vi "AlGaInPAs_v20a.vi"(2 "Debug Mode":bool, 3 "Elapsed Time(s)":dbl, 4 "State":enum16{"Edit", "Start", "Run", "End", "Idle"}(ring), 5 "Argument List In":string[](array[string])) -> (0 "Status Out":string, 1 "Argument List Out":string[](array[string]))   [LabVIEW 2011]
uses:
  high_level_proc/Al_bubbler.ctl
  high_level_proc/bubblerDilution.ctl
  high_level_proc/In_bubbler.ctl
  high_level_proc/P_gas.ctl
  high_level_proc/As_gas.ctl
  high_level_proc/P_bubbler.ctl
panel:
  out "Se bubbler Copy":T1={"Active"=FALSE, "main"={"Flow"=0.0, "Run"=FALSE, "Prep Ga"=FALSE, "Dilution"=FALSE, "Calculated"=1, "MFC2 flow"=10.0, "MFC3 flow"=100.0, "MFC1 flow"=0.0}} {"main"."MFC1 flow" format="%.4f"; "main"."MFC3 flow" format="%.1f"; "main"."MFC2 flow" format="%.2f"; "main"."Calculated" items=["Ga flow", "MFC1", "MFC2", "MFC3"]; "main"."Flow" format="%.2f"}
  in  "Se bubbler":T1={"Active"=FALSE, "main"={"Flow"=0.0, "Run"=FALSE, "Prep Ga"=FALSE, "Dilution"=FALSE, "Calculated"=0, "MFC2 flow"=10.0, "MFC3 flow"=100.0, "MFC1 flow"=0.0}} {"main"."MFC1 flow" format="%.4f"; "main"."MFC3 flow" format="%.1f"; "main"."MFC2 flow" format="%.2f"; "main"."Calculated" items=["Flow", "MFC1", "MFC2", "MFC3"]; "main"."Flow" format="%.2f"}
  out "P bubbler Copy":T2 {"P bubbler main"."Flow" format="%.2f"}
  in  "P bubbler":T3 {"P bubbler main"."Flow" format="%.2f"}
  out "As gas Copy":T4 {"As gas main"."Flow" format="%.2f"}
  in  "As gas":T5 {"As gas main"."Flow" format="%.2f"}
  out "P gas Copy":T6 {"P gas main"."Flow" format="%.2f"}
  in  "P gas":T7 {"P gas main"."Flow" format="%.2f"}
  out "In bubbler Copy":T8 {"In main"."Flow" format="%.2f"}
  in  "In bubbler":T9 {"In main"."Flow" format="%.2f"}
  out "Ga bubbler Copy":T10={"Ga bubbler Active"=FALSE, "Ga main"={"Flow"=0.0, "Ga Run"=FALSE, "Prep Ga"=FALSE, "Dilution"=FALSE, "Ga Calculated"=1, "MFC2 flow"=10.0, "MFC3 flow"=100.0, "MFC1 flow"=0.0}} {"Ga main"."MFC1 flow" format="%.4f"; "Ga main"."MFC3 flow" format="%.1f"; "Ga main"."MFC2 flow" format="%.2f"; "Ga main"."Ga Calculated" items=["Ga flow", "MFC1", "MFC2", "MFC3"]; "Ga main"."Flow" format="%.2f"}
  in  "Ga bubbler":T1={"Active"=FALSE, "main"={"Flow"=0.0, "Run"=FALSE, "Prep Ga"=FALSE, "Dilution"=FALSE, "Calculated"=0, "MFC2 flow"=10.0, "MFC3 flow"=100.0, "MFC1 flow"=0.0}} {"main"."MFC1 flow" format="%.4f"; "main"."MFC3 flow" format="%.1f"; "main"."MFC2 flow" format="%.2f"; "main"."Calculated" items=["Flow", "MFC1", "MFC2", "MFC3"]; "main"."Flow" format="%.2f"}
  out "Al bubbler Copy":T11 {"Al main"."Al Flow" format="%.2f"}
  in  "Al bubbler":T12 {"Al main"."Al Flow" format="%.2f"}
  out "prep_done":bool
  out "run started":bool
  out "first":bool=TRUE
  out "total time":dbl
  out "is OK?":bool
  in  "prep_time":dbl
  in  "Cancel":bool
  in  "OK":bool
  out "tTotal(s) 2":dbl
  # "s"
  # "Add pre-run time to run time in editor."
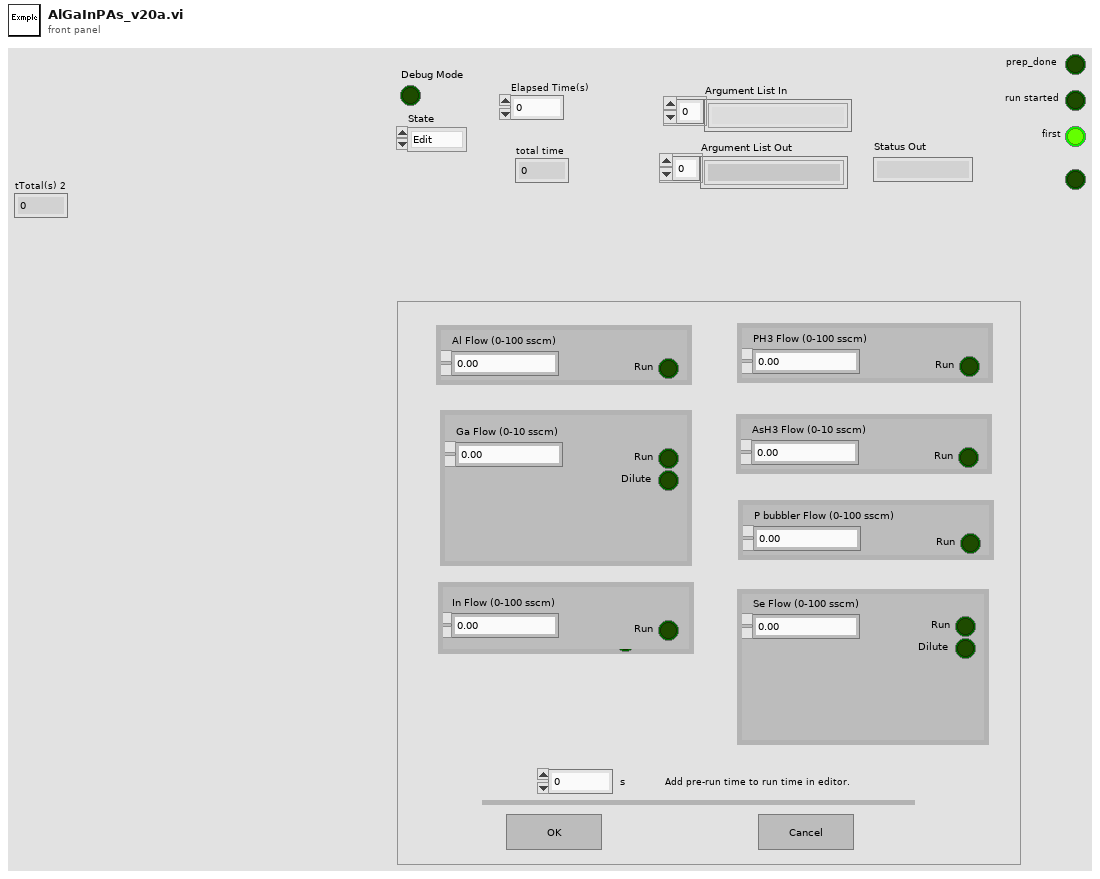
[diagram p1: front panel]
types:
  T1 = typedef "bubblerDilution.ctl" = cluster{"Active":bool, "main":cluster{"Flow":dbl, "Run":bool, "Prep Ga":bool, "Dilution":bool, "Calculated":u16, "MFC2 flow":dbl, "MFC3 flow":dbl, "MFC1 flow":dbl}}
  T2 = cluster{"P bubbler Active":bool, "P bubbler main":cluster{"Flow":dbl, "P bubbler Run":bool, "P bubbler Prep":bool}}
  T3 = typedef "P_bubbler.ctl" = cluster{"P bubbler Active":bool, "P bubbler main":cluster{"Flow":dbl, "P bubbler Run":bool, "P bubbler Prep":bool}}
  T4 = cluster{"As gas Active":bool, "As gas main":cluster{"Flow":dbl, "AsH3 Run":bool, "AsH3 Prep":bool}}
  T5 = typedef "As_gas.ctl" = cluster{"As gas Active":bool, "As gas main":cluster{"Flow":dbl, "AsH3 Run":bool, "AsH3 Prep":bool}}
  T6 = cluster{"P gas Active":bool, "P gas main":cluster{"Flow":dbl, "PH3 Run":bool, "PH3 Prep":bool}}
  T7 = typedef "P_gas.ctl" = cluster{"P gas Active":bool, "P gas main":cluster{"Flow":dbl, "PH3 Run":bool, "PH3 Prep":bool}}
  T8 = cluster{"In main":cluster{"Flow":dbl, "In Run":bool, "Prep In":bool}, "In bubbler Active":bool}
  T9 = typedef "In_bubbler.ctl" = cluster{"In main":cluster{"Flow":dbl, "In Run":bool, "Prep In":bool}, "In bubbler Active":bool}
  T10 = cluster{"Ga bubbler Active":bool, "Ga main":cluster{"Flow":dbl, "Ga Run":bool, "Prep Ga":bool, "Dilution":bool, "Ga Calculated":u16, "MFC2 flow":dbl, "MFC3 flow":dbl, "MFC1 flow":dbl}}
  T11 = cluster{"Al Active":bool, "Al main":cluster{"Al Flow":dbl, "Al Run":bool, "Prep Al":bool}}
  T12 = typedef "Al_bubbler.ctl" = cluster{"Al Active":bool, "Al main":cluster{"Al Flow":dbl, "Al Run":bool, "Prep Al":bool}}
  T13 = enum16{"Discrete", "Continuous", "Instantaneous", "Finite"}
  T14 = enum32{"Invalid", "Default", "Floating", "Floating/Auto-Hide", "Modal"}
  T15 = enum8{"Enabled", "Disabled", "Disabled and Grayed Out"}
  T16 = cluster{"Active":bool, "main":cluster{"Flow":dbl, "Run":bool, "Prep Ga":bool, "Dilution":bool, "Calculated":u16, "MFC2 flow":dbl, "MFC3 flow":dbl, "MFC1 flow":dbl}}
  T17 = cluster{"Al Flow":dbl, "Al Run":bool, "Prep Al":bool}
  T18 = cluster{"Flow":dbl, "Run":bool, "Prep Ga":bool, "Dilution":bool, "Calculated":u16, "MFC2 flow":dbl, "MFC3 flow":dbl, "MFC1 flow":dbl}
  T19 = cluster{"Flow":dbl, "In Run":bool, "Prep In":bool}
  T20 = cluster{"Flow":dbl, "PH3 Run":bool, "PH3 Prep":bool}
  T21 = cluster{"Flow":dbl, "AsH3 Run":bool, "AsH3 Prep":bool}
  T22 = cluster{"Flow":dbl, "P bubbler Run":bool, "P bubbler Prep":bool}
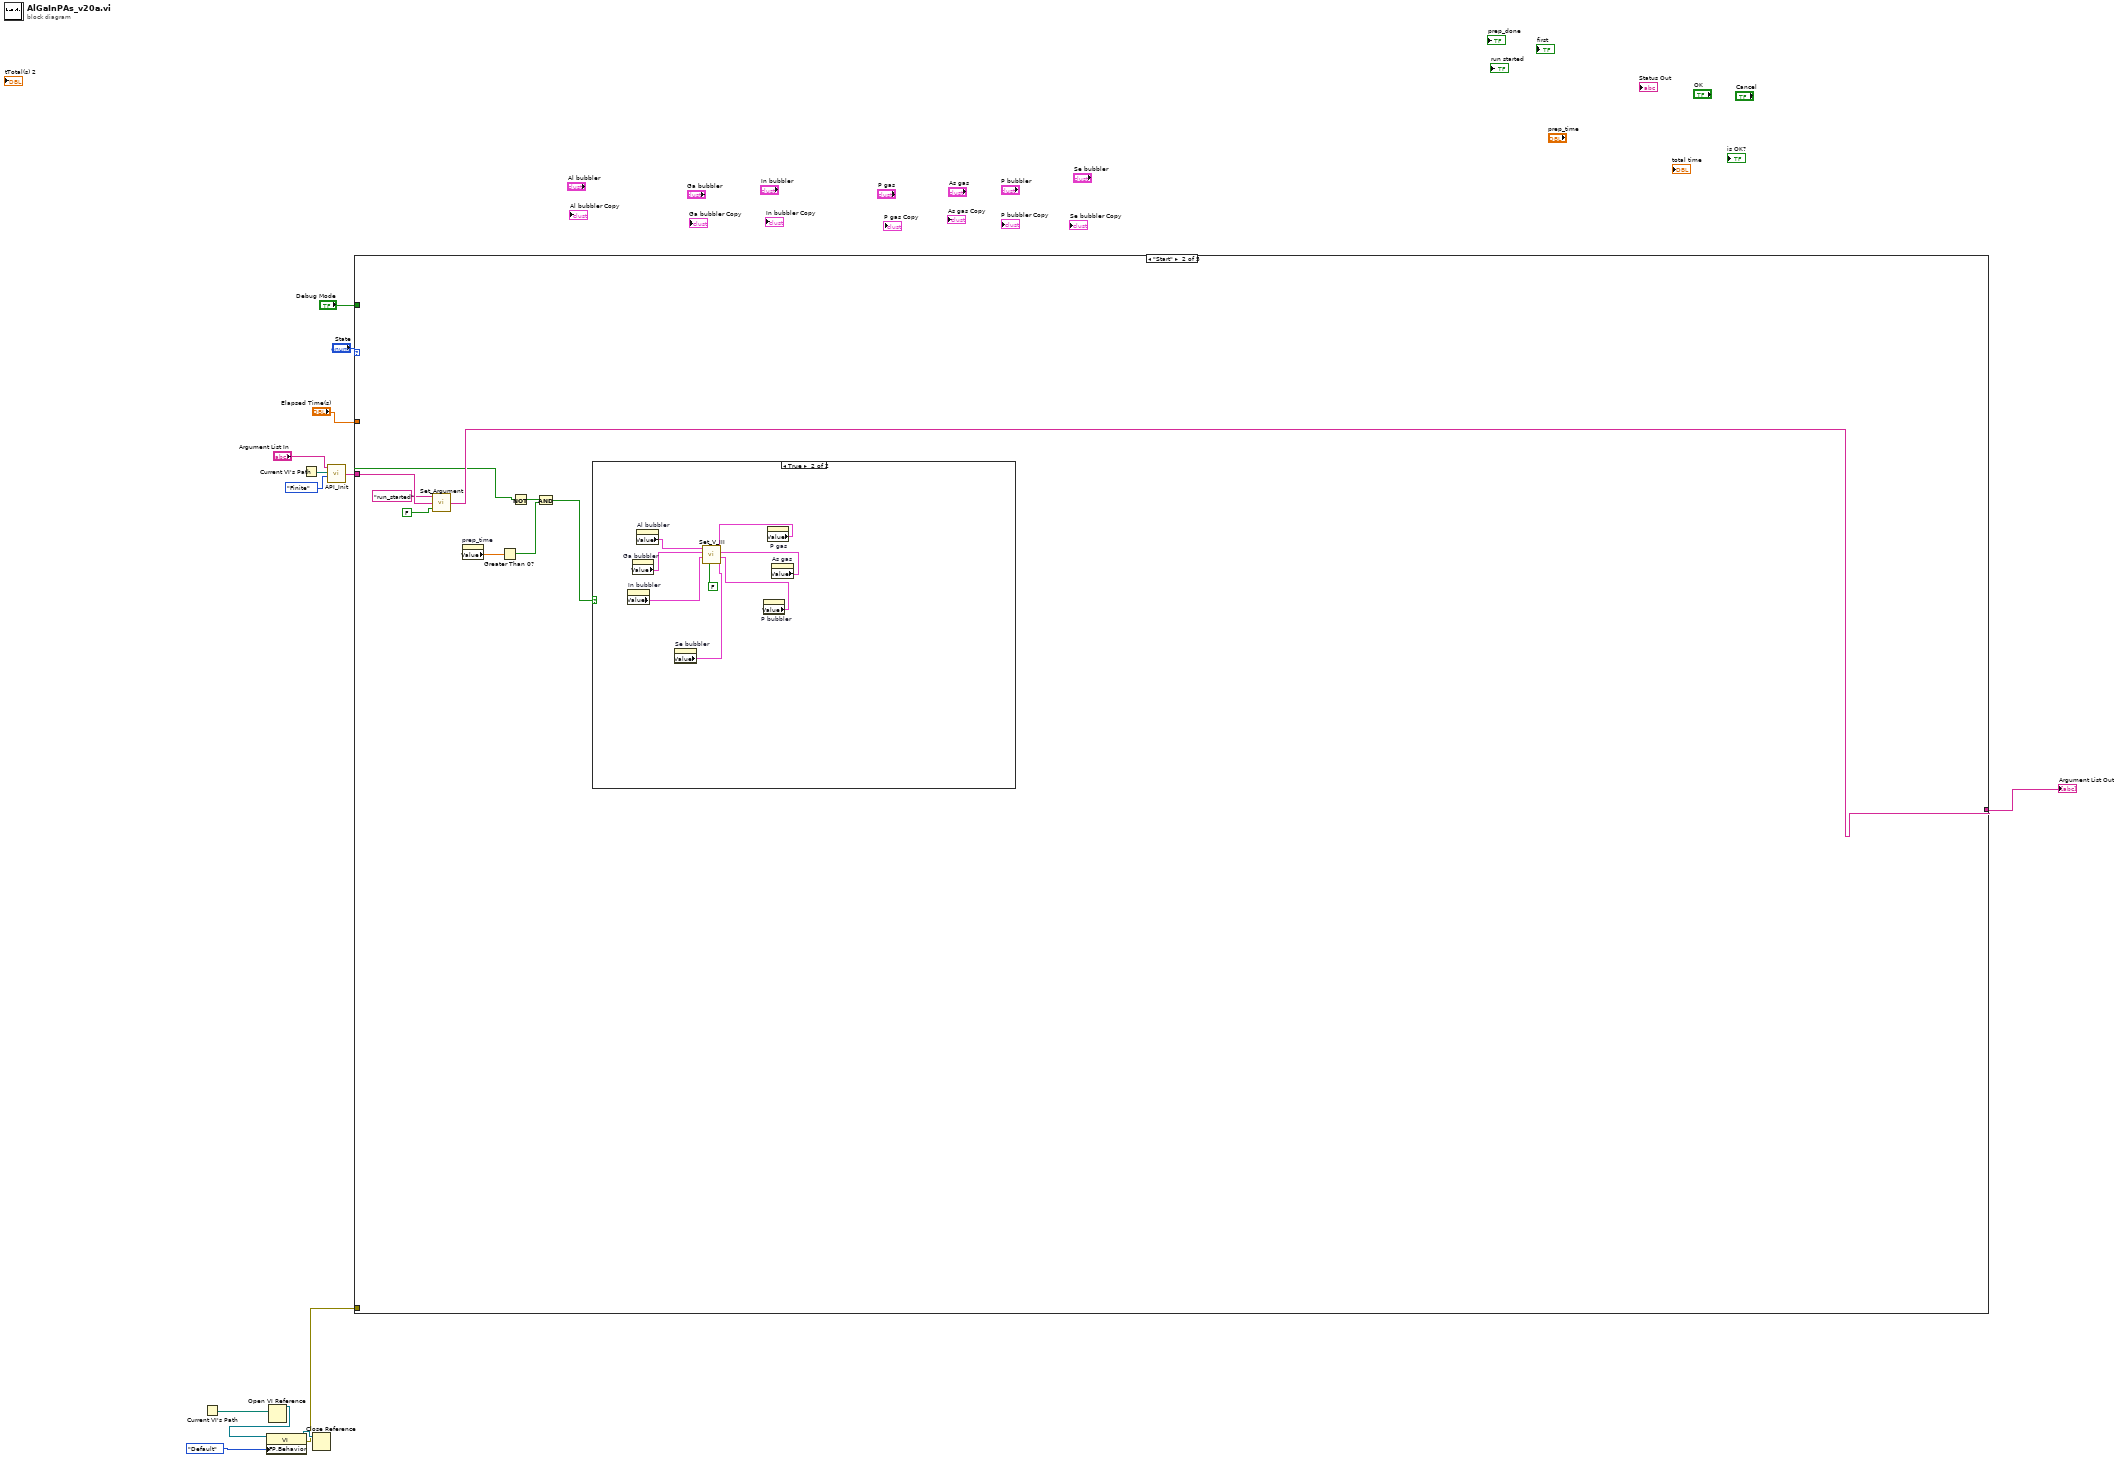
[diagram p0: block diagram]
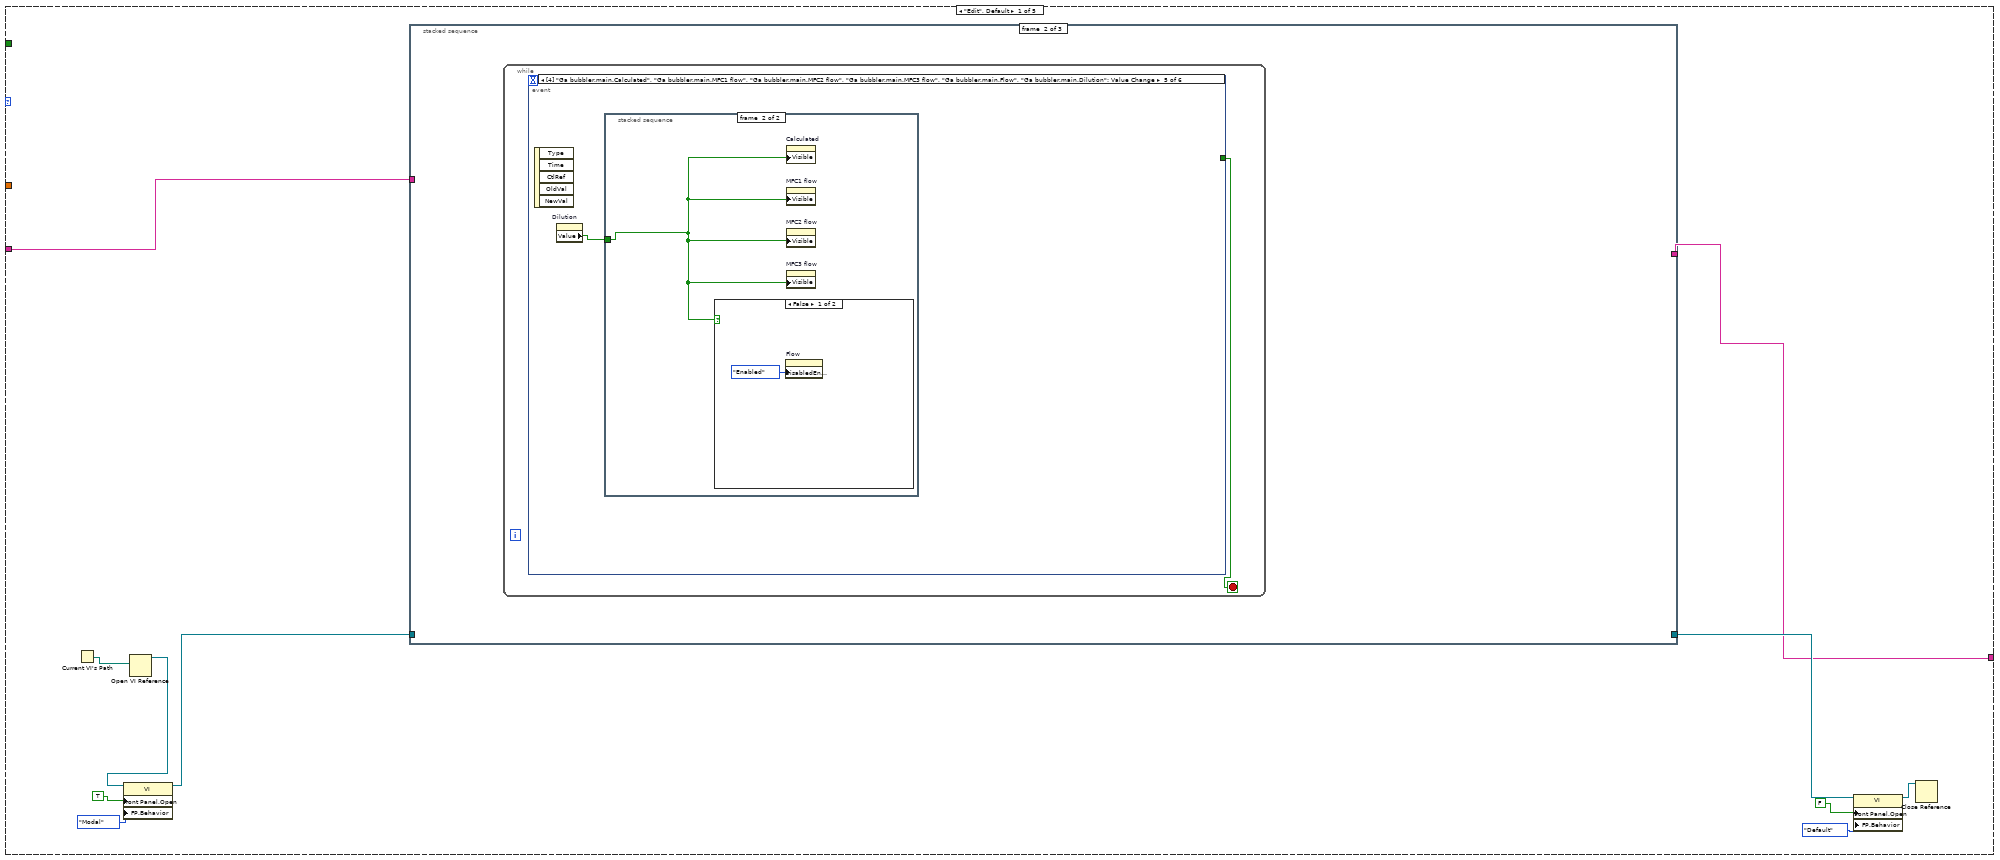
[diagram p2: hidden frame]
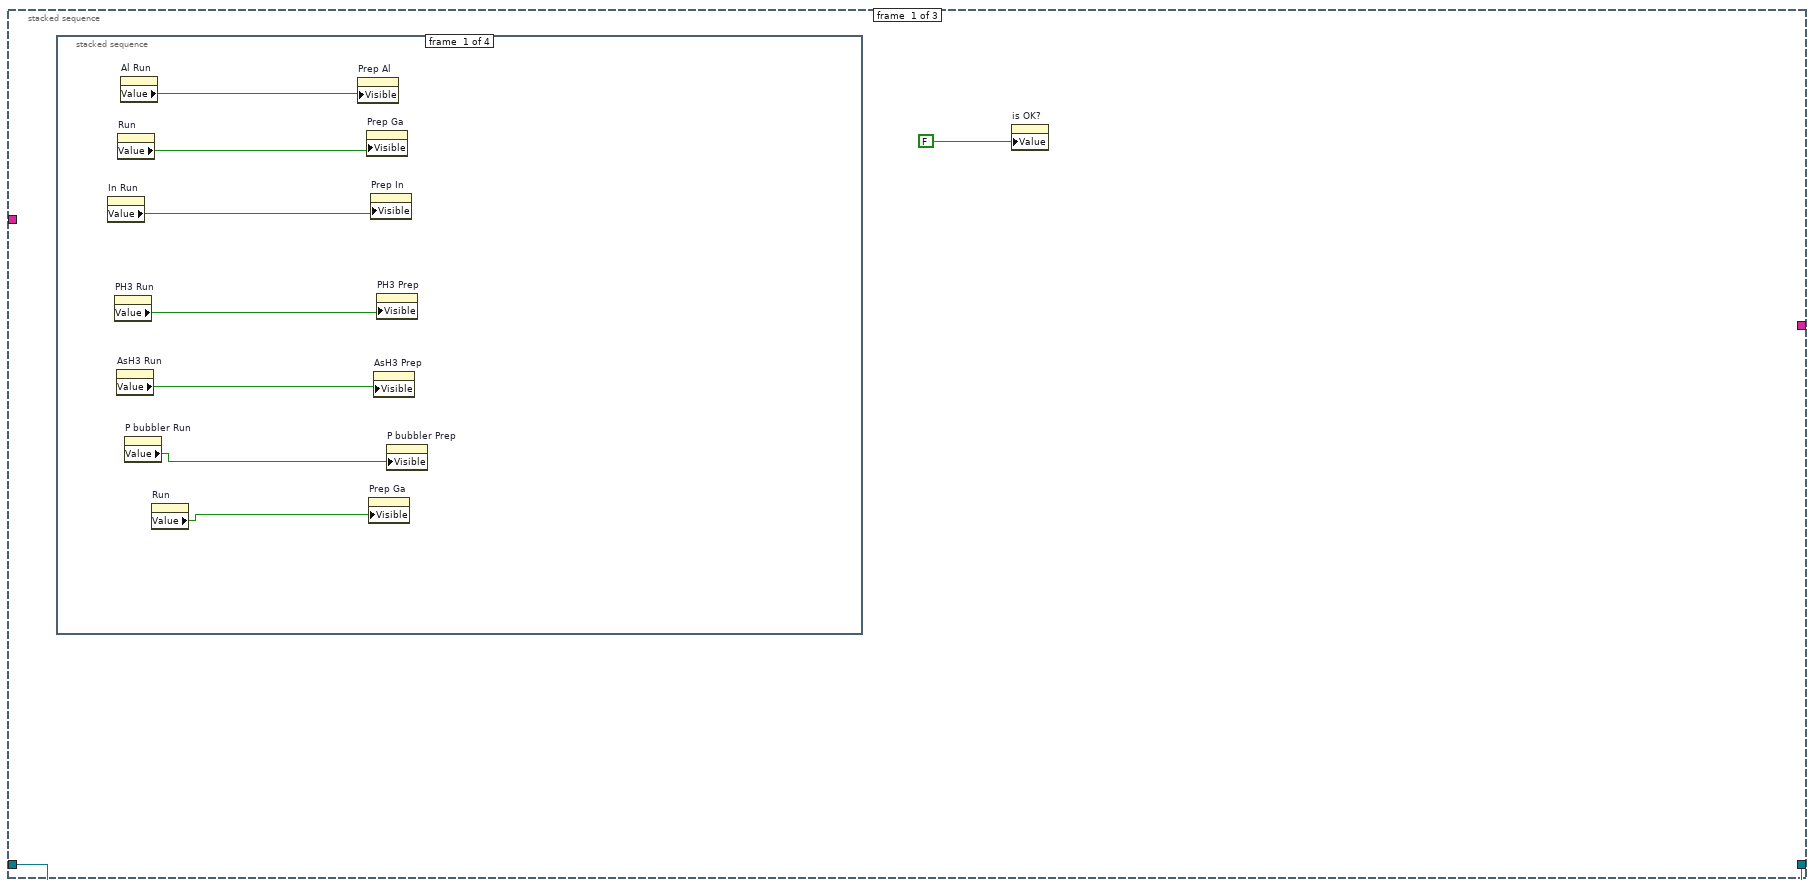
[diagram p3: hidden frame]
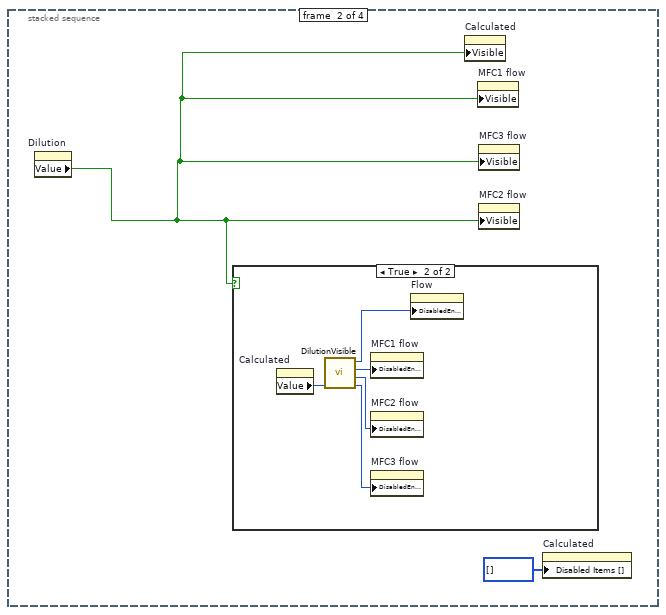
[diagram p4: hidden frame]
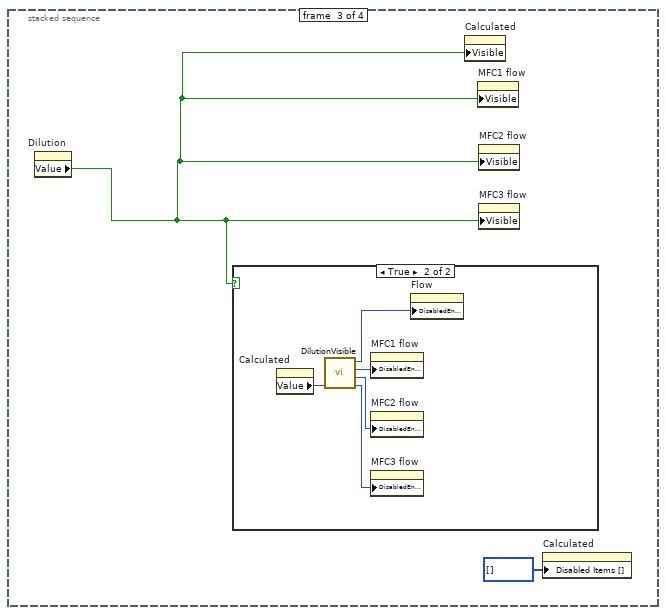
[diagram p6: hidden frame]
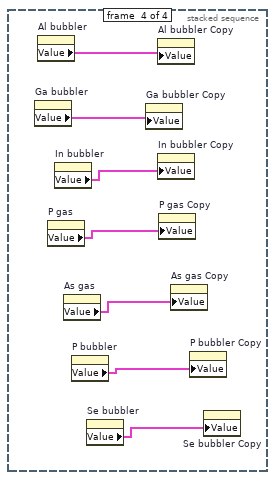
[diagram p8: hidden frame]
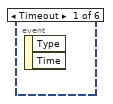
[diagram p9: hidden frame]
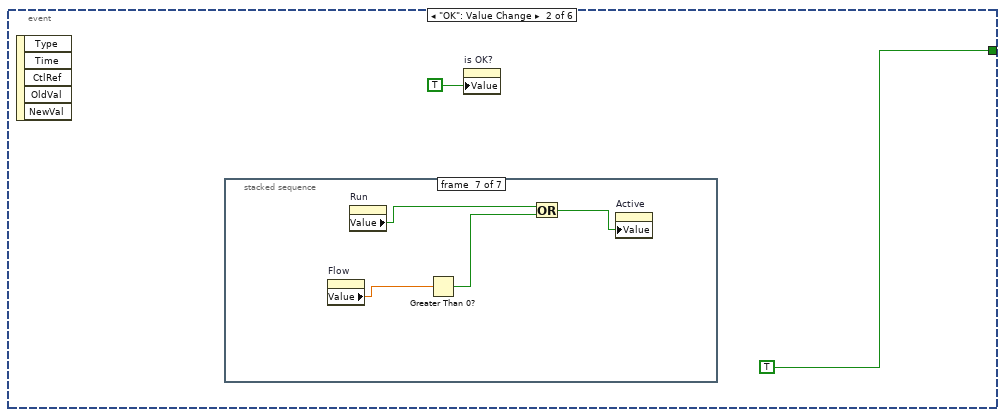
[diagram p10: hidden frame]
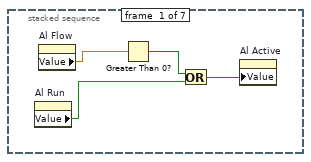
[diagram p11: hidden frame]
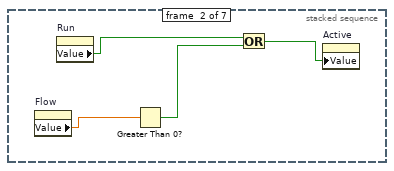
[diagram p12: hidden frame]
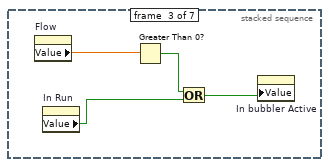
[diagram p13: hidden frame]
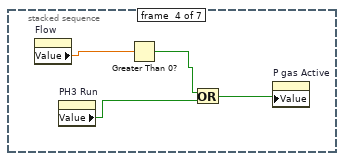
[diagram p14: hidden frame]
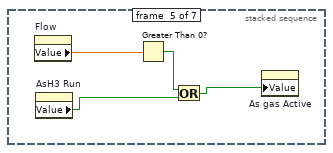
[diagram p15: hidden frame]
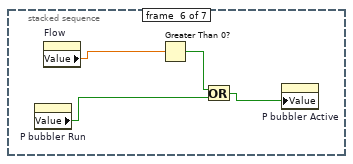
[diagram p16: hidden frame]
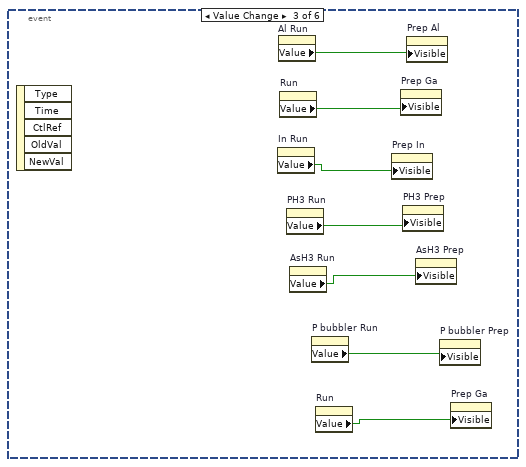
[diagram p17: hidden frame]
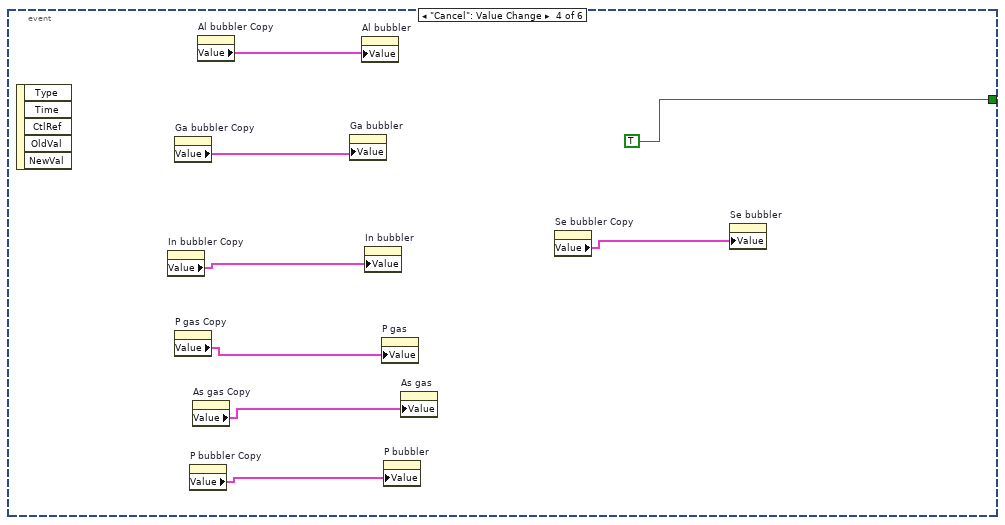
[diagram p18: hidden frame]
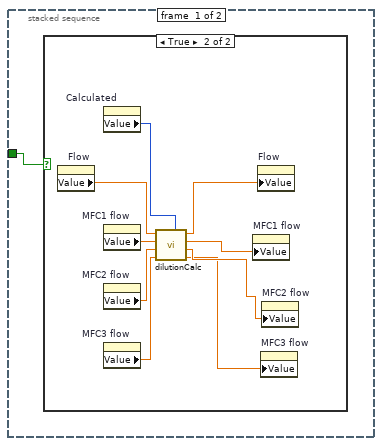
[diagram p19: hidden frame]
diagram:
  n1 = Current VI's Path() -> (path=w9:path)
  n2 = Open VI Reference(vi path=w9) -> (vi reference=w8:refnum<vi>)  [unwired: 1 in, 5 out]
  n3 = property class="VI"(reference=w8, "FP.Behavior"=T14."Default" ("Front Panel Window:Behavior")) -> (reference out=w6:refnum<vi>, error out=w5:errorcluster)  [unwired: 1 in]
  n4 = Current VI's Path() -> (path=w4:path)
  n5 = Close Reference(reference=w6) -> ()  [unwired: 1 in, 1 out]
  n6 = call "API_Init.vi"("API Mode"=T13."Finite", "VI Path"=w4, "Argument List In"="Argument List In") -> ("Argument List Out"=w1:string[])  [unwired: 1 in]
  n7 = case shown="\"Start\"" "State" {
    tunnel: "Debug Mode" -> [_ w143 w161 _ _]
    tunnel: "Elapsed Time(s)" -> [_ _ w162 _ _]
    tunnel: w1 -> [w15 w148 w160 w271 w272]
    tunnel: [w14 w147 w159 w271 w272] -> w10
    tunnel: w5 -> [_ _ _ _ _]
    frame "Edit", Default {
      n8 = Current VI's Path() -> (path=w20:path)
      n9 = Open VI Reference(vi path=w20) -> (vi reference=w19:refnum<vi>)  [unwired: 1 in, 5 out]
      n10 = property class="VI"(reference=w19, "Front Panel.Open"=TRUE ("Front Panel Window:Open"), "FP.Behavior"=T14."Modal" ("Front Panel Window:Behavior")) -> (reference out=w18:refnum<vi>)  [unwired: 1 in, 1 out]
      n11 = stacked-sequence {
        tunnel: w15 -> [_ _ w138]
        tunnel: w18 -> [w26 _ _]
        tunnel: [w26 _ _] -> w22
        tunnel: [_ _ w139] -> w14
        frame #0 {
          n12 = stacked-sequence {
            frame #0 {
              n13 = property on="In Run" class="Bool (strict)"() -> ("Value"=w32:bool)  [unwired: 2 in, 2 out]
              n14 = property on="PH3 Run" class="Bool (strict)"() -> ("Value"=w30:bool)  [unwired: 2 in, 2 out]
              n15 = property on="AsH3 Run" class="Bool (strict)"() -> ("Value"=w29:bool)  [unwired: 2 in, 2 out]
              n16 = property on="Run" class="Bool (strict)"() -> ("Value"=w31:bool)  [unwired: 2 in, 2 out]
              n17 = property on="Al Run" class="Bool (strict)"() -> ("Value"=w33:bool)  [unwired: 2 in, 2 out]
              n18 = property on="P bubbler Run" class="Bool (strict)"() -> ("Value"=w28:bool)  [unwired: 2 in, 2 out]
              n19 = property on="Run" class="Bool (strict)"() -> ("Value"=w27:bool)  [unwired: 2 in, 2 out]
              n20 = property on="Prep Al" class="Bool (strict)"("Visible"=w33) -> ()  [unwired: 2 in, 2 out]
              n21 = property on="Prep Ga" class="Bool (strict)"("Visible"=w31) -> ()  [unwired: 2 in, 2 out]
              n22 = property on="Prep Ga" class="Bool (strict)"("Visible"=w27) -> ()  [unwired: 2 in, 2 out]
              n23 = property on="Prep In" class="Bool (strict)"("Visible"=w32) -> ()  [unwired: 2 in, 2 out]
              n24 = property on="AsH3 Prep" class="Bool (strict)"("Visible"=w29) -> ()  [unwired: 2 in, 2 out]
              n25 = property on="PH3 Prep" class="Bool (strict)"("Visible"=w30) -> ()  [unwired: 2 in, 2 out]
              n26 = property on="P bubbler Prep" class="Bool (strict)"("Visible"=w28) -> ()  [unwired: 2 in, 2 out]
            }
            frame #1 {
              n27 = property on="Dilution" class="Bool (strict)"() -> ("Value"=w35:bool)  [unwired: 2 in, 2 out]
              n28 = case shown="True" w35 {
                frame False {
                }
                frame True {
                  n29 = property on="Calculated" class="Ring (strict)"() -> ("Value"=w36:u16)  [unwired: 2 in, 2 out]
                  n30 = call "DilutionVisible.vi"("calculated"=w36) -> ("MFC3"=w39:u16, "MFC2"=w38:u16, "MFC1"=w37:u16, "flow"=w40:u16)  [unwired: 3 in]
                  n31 = property on="MFC1 flow" class="DigNum (strict)"("DisabledEnum"=w37) -> ()  [unwired: 2 in, 2 out]
                  n32 = property on="MFC2 flow" class="DigNum (strict)"("DisabledEnum"=w38) -> ()  [unwired: 2 in, 2 out]
                  n33 = property on="MFC3 flow" class="DigNum (strict)"("DisabledEnum"=w39) -> ()  [unwired: 2 in, 2 out]
                  n34 = property on="Flow" class="DigNum (strict)"("DisabledEnum"=w40) -> ()  [unwired: 2 in, 2 out]
                }
              }
              n35 = property on="Calculated" class="Ring (strict)"("Visible"=w35) -> ()  [unwired: 2 in, 2 out]
              n36 = property on="MFC1 flow" class="DigNum (strict)"("Visible"=w35) -> ()  [unwired: 2 in, 2 out]
              n37 = property on="MFC3 flow" class="DigNum (strict)"("Visible"=w35) -> ()  [unwired: 2 in, 2 out]
              n38 = property on="MFC2 flow" class="DigNum (strict)"("Visible"=w35) -> ()  [unwired: 2 in, 2 out]
              n39 = property on="Calculated" class="Ring (strict)"("Disabled Items []"=i32[] []) -> ()  [unwired: 2 in, 2 out]
            }
            frame #2 {
              n40 = property on="Dilution" class="Bool (strict)"() -> ("Value"=w42:bool)  [unwired: 2 in, 2 out]
              n41 = case shown="True" w42 {
                frame False {
                }
                frame True {
                  n42 = property on="Calculated" class="Ring (strict)"() -> ("Value"=w43:u16)  [unwired: 2 in, 2 out]
                  n43 = call "DilutionVisible.vi"("calculated"=w43) -> ("MFC3"=w46:u16, "MFC2"=w45:u16, "MFC1"=w44:u16, "flow"=w47:u16)  [unwired: 3 in]
                  n44 = property on="MFC1 flow" class="DigNum (strict)"("DisabledEnum"=w44) -> ()  [unwired: 2 in, 2 out]
                  n45 = property on="MFC2 flow" class="DigNum (strict)"("DisabledEnum"=w45) -> ()  [unwired: 2 in, 2 out]
                  n46 = property on="MFC3 flow" class="DigNum (strict)"("DisabledEnum"=w46) -> ()  [unwired: 2 in, 2 out]
                  n47 = property on="Flow" class="DigNum (strict)"("DisabledEnum"=w47) -> ()  [unwired: 2 in, 2 out]
                }
              }
              n48 = property on="Calculated" class="Ring (strict)"("Visible"=w42) -> ()  [unwired: 2 in, 2 out]
              n49 = property on="MFC1 flow" class="DigNum (strict)"("Visible"=w42) -> ()  [unwired: 2 in, 2 out]
              n50 = property on="MFC2 flow" class="DigNum (strict)"("Visible"=w42) -> ()  [unwired: 2 in, 2 out]
              n51 = property on="MFC3 flow" class="DigNum (strict)"("Visible"=w42) -> ()  [unwired: 2 in, 2 out]
              n52 = property on="Calculated" class="Ring (strict)"("Disabled Items []"=i32[] []) -> ()  [unwired: 2 in, 2 out]
            }
            frame #3 {
              n53 = property on="Ga bubbler" class="Clust (strict)"() -> ("Value"=w53:T16)  [unwired: 2 in, 2 out]
              n54 = property on="Al bubbler" class="Clust (strict)"() -> ("Value"=w54:T11)  [unwired: 2 in, 2 out]
              n55 = property on="P gas" class="Clust (strict)"() -> ("Value"=w51:T6)  [unwired: 2 in, 2 out]
              n56 = property on="In bubbler" class="Clust (strict)"() -> ("Value"=w52:T8)  [unwired: 2 in, 2 out]
              n57 = property on="As gas" class="Clust (strict)"() -> ("Value"=w50:T4)  [unwired: 2 in, 2 out]
              n58 = property on="P bubbler" class="Clust (strict)"() -> ("Value"=w49:T2)  [unwired: 2 in, 2 out]
              n59 = property on="Se bubbler" class="Clust (strict)"() -> ("Value"=w48:T16)  [unwired: 2 in, 2 out]
              n60 = property on="Ga bubbler Copy" class="Clust (strict)"("Value"=w53) -> ()  [unwired: 2 in, 2 out]
              n61 = property on="Al bubbler Copy" class="Clust (strict)"("Value"=w54) -> ()  [unwired: 2 in, 2 out]
              n62 = property on="In bubbler Copy" class="Clust (strict)"("Value"=w52) -> ()  [unwired: 2 in, 2 out]
              n63 = property on="P gas Copy" class="Clust (strict)"("Value"=w51) -> ()  [unwired: 2 in, 2 out]
              n64 = property on="As gas Copy" class="Clust (strict)"("Value"=w50) -> ()  [unwired: 2 in, 2 out]
              n65 = property on="P bubbler Copy" class="Clust (strict)"("Value"=w49) -> ()  [unwired: 2 in, 2 out]
              n66 = property on="Se bubbler Copy" class="Clust (strict)"("Value"=w48) -> ()  [unwired: 2 in, 2 out]
            }
          }
          n67 = property on="is OK?" class="Bool (strict)"("Value"=FALSE ("is OK?")) -> ()  [unwired: 2 in, 2 out]
        }
        frame #1 {
          n68 = while {
            stop <- w55 stop-if-true
            n69 = event shown="[4] \"Ga bubbler.main.Calculated\", \"Ga bubbler.main.MFC1 flow\", \"Ga bubbler.main.MFC2 flow\", \"Ga bubbler.main.MFC3 flow\", \"Ga bubbler.main.Flow\", \"Ga bubbler.main.Dilution\": Value Change" {
              selector: _ -> [_ _ _ _ _ _]
              dyn-events: _ -> [_ _ _ _ _ _]
              timeout: _ -> [_ _ _ _ _ _]
              tunnel: [_ TRUE _ TRUE _ _] -> w55
              event Timeout {
                n70 = event-data() -> ()  [unwired: 1 in, 2 out]
              }
              event "OK": Value Change {
                n71 = event-data() -> ()  [unwired: 1 in, 5 out]
                n72 = stacked-sequence {
                  frame #0 {
                    n73 = property on="Al Run" class="Bool (strict)"() -> ("Value"=w59:bool)  [unwired: 2 in, 2 out]
                    n74 = property on="Al Flow" class="DigNum (strict)"() -> ("Value"=w60:dbl)  [unwired: 2 in, 2 out]
                    n75 = Greater Than 0?(x=w60) -> (x > 0?=w61:bool)
                    n76 = Or(x=w61, y=w59) -> (x .or. y?=w58:bool)
                    n77 = property on="Al Active" class="Bool (strict)"("Value"=w58) -> ()  [unwired: 2 in, 2 out]
                  }
                  frame #1 {
                    n78 = property on="Flow" class="DigNum (strict)"() -> ("Value"=w62:dbl)  [unwired: 2 in, 2 out]
                    n79 = property on="Run" class="Bool (strict)"() -> ("Value"=w63:bool)  [unwired: 2 in, 2 out]
                    n80 = Greater Than 0?(x=w62) -> (x > 0?=w65:bool)
                    n81 = Or(x=w63, y=w65) -> (x .or. y?=w64:bool)
                    n82 = property on="Active" class="Bool (strict)"("Value"=w64) -> ()  [unwired: 2 in, 2 out]
                  }
                  frame #2 {
                    n83 = property on="Flow" class="DigNum (strict)"() -> ("Value"=w68:dbl)  [unwired: 2 in, 2 out]
                    n84 = property on="In Run" class="Bool (strict)"() -> ("Value"=w67:bool)  [unwired: 2 in, 2 out]
                    n85 = Greater Than 0?(x=w68) -> (x > 0?=w69:bool)
                    n86 = Or(x=w69, y=w67) -> (x .or. y?=w66:bool)
                    n87 = property on="In bubbler Active" class="Bool (strict)"("Value"=w66) -> ()  [unwired: 2 in, 2 out]
                  }
                  frame #3 {
                    n88 = property on="Flow" class="DigNum (strict)"() -> ("Value"=w72:dbl)  [unwired: 2 in, 2 out]
                    n89 = property on="PH3 Run" class="Bool (strict)"() -> ("Value"=w71:bool)  [unwired: 2 in, 2 out]
                    n90 = Greater Than 0?(x=w72) -> (x > 0?=w73:bool)
                    n91 = Or(x=w73, y=w71) -> (x .or. y?=w70:bool)
                    n92 = property on="P gas Active" class="Bool (strict)"("Value"=w70) -> ()  [unwired: 2 in, 2 out]
                  }
                  frame #4 {
                    n93 = property on="Flow" class="DigNum (strict)"() -> ("Value"=w76:dbl)  [unwired: 2 in, 2 out]
                    n94 = property on="AsH3 Run" class="Bool (strict)"() -> ("Value"=w75:bool)  [unwired: 2 in, 2 out]
                    n95 = Greater Than 0?(x=w76) -> (x > 0?=w77:bool)
                    n96 = Or(x=w77, y=w75) -> (x .or. y?=w74:bool)
                    n97 = property on="As gas Active" class="Bool (strict)"("Value"=w74) -> ()  [unwired: 2 in, 2 out]
                  }
                  frame #5 {
                    n98 = property on="P bubbler Run" class="Bool (strict)"() -> ("Value"=w79:bool)  [unwired: 2 in, 2 out]
                    n99 = property on="Flow" class="DigNum (strict)"() -> ("Value"=w80:dbl)  [unwired: 2 in, 2 out]
                    n100 = Greater Than 0?(x=w80) -> (x > 0?=w81:bool)
                    n101 = Or(x=w81, y=w79) -> (x .or. y?=w78:bool)
                    n102 = property on="P bubbler Active" class="Bool (strict)"("Value"=w78) -> ()  [unwired: 2 in, 2 out]
                  }
                  frame #6 {
                    n103 = property on="Flow" class="DigNum (strict)"() -> ("Value"=w82:dbl)  [unwired: 2 in, 2 out]
                    n104 = property on="Run" class="Bool (strict)"() -> ("Value"=w83:bool)  [unwired: 2 in, 2 out]
                    n105 = Greater Than 0?(x=w82) -> (x > 0?=w85:bool)
                    n106 = Or(x=w83, y=w85) -> (x .or. y?=w84:bool)
                    n107 = property on="Active" class="Bool (strict)"("Value"=w84) -> ()  [unwired: 2 in, 2 out]
                  }
                }
                n108 = property on="is OK?" class="Bool (strict)"("Value"=TRUE ("is OK?")) -> ()  [unwired: 2 in, 2 out]
              }
              event Value Change {
                n109 = event-data() -> ()  [unwired: 1 in, 5 out]
                n110 = property on="In Run" class="Bool (strict)"() -> ("Value"=w89:bool)  [unwired: 2 in, 2 out]
                n111 = property on="Al Run" class="Bool (strict)"() -> ("Value"=w91:bool)  [unwired: 2 in, 2 out]
                n112 = property on="Run" class="Bool (strict)"() -> ("Value"=w90:bool)  [unwired: 2 in, 2 out]
                n113 = property on="PH3 Run" class="Bool (strict)"() -> ("Value"=w88:bool)  [unwired: 2 in, 2 out]
                n114 = property on="AsH3 Run" class="Bool (strict)"() -> ("Value"=w87:bool)  [unwired: 2 in, 2 out]
                n115 = property on="P bubbler Run" class="Bool (strict)"() -> ("Value"=w92:bool)  [unwired: 2 in, 2 out]
                n116 = property on="Run" class="Bool (strict)"() -> ("Value"=w86:bool)  [unwired: 2 in, 2 out]
                n117 = property on="Prep In" class="Bool (strict)"("Visible"=w89) -> ()  [unwired: 2 in, 2 out]
                n118 = property on="Prep Ga" class="Bool (strict)"("Visible"=w90) -> ()  [unwired: 2 in, 2 out]
                n119 = property on="PH3 Prep" class="Bool (strict)"("Visible"=w88) -> ()  [unwired: 2 in, 2 out]
                n120 = property on="Prep Al" class="Bool (strict)"("Visible"=w91) -> ()  [unwired: 2 in, 2 out]
                n121 = property on="AsH3 Prep" class="Bool (strict)"("Visible"=w87) -> ()  [unwired: 2 in, 2 out]
                n122 = property on="P bubbler Prep" class="Bool (strict)"("Visible"=w92) -> ()  [unwired: 2 in, 2 out]
                n123 = property on="Prep Ga" class="Bool (strict)"("Visible"=w86) -> ()  [unwired: 2 in, 2 out]
              }
              event "Cancel": Value Change {
                n124 = event-data() -> ()  [unwired: 1 in, 5 out]
                n125 = property on="In bubbler Copy" class="Clust (strict)"() -> ("Value"=w98:T8)  [unwired: 2 in, 2 out]
                n126 = property on="Ga bubbler Copy" class="Clust (strict)"() -> ("Value"=w97:T10)  [unwired: 2 in, 2 out]
                n127 = property on="P gas Copy" class="Clust (strict)"() -> ("Value"=w96:T6)  [unwired: 2 in, 2 out]
                n128 = property on="P bubbler Copy" class="Clust (strict)"() -> ("Value"=w94:T2)  [unwired: 2 in, 2 out]
                n129 = property on="As gas Copy" class="Clust (strict)"() -> ("Value"=w95:T4)  [unwired: 2 in, 2 out]
                n130 = property on="Al bubbler Copy" class="Clust (strict)"() -> ("Value"=w99:T11)  [unwired: 2 in, 2 out]
                n131 = property on="Ga bubbler" class="Clust (strict)"("Value"=w97) -> ()  [unwired: 2 in, 2 out]
                n132 = property on="Al bubbler" class="Clust (strict)"("Value"=w99) -> ()  [unwired: 2 in, 2 out]
                n133 = property on="In bubbler" class="Clust (strict)"("Value"=w98) -> ()  [unwired: 2 in, 2 out]
                n134 = property on="P gas" class="Clust (strict)"("Value"=w96) -> ()  [unwired: 2 in, 2 out]
                n135 = property on="P bubbler" class="Clust (strict)"("Value"=w94) -> ()  [unwired: 2 in, 2 out]
                n136 = property on="As gas" class="Clust (strict)"("Value"=w95) -> ()  [unwired: 2 in, 2 out]
                n137 = property on="Se bubbler Copy" class="Clust (strict)"() -> ("Value"=w93:T16)  [unwired: 2 in, 2 out]
                n138 = property on="Se bubbler" class="Clust (strict)"("Value"=w93) -> ()  [unwired: 2 in, 2 out]
              }
              event Value Change {
                n139 = event-data() -> ()  [unwired: 1 in, 5 out]
                n140 = property on="Dilution" class="Bool (strict)"() -> ("Value"=w101:bool)  [unwired: 2 in, 2 out]
                n141 = stacked-sequence {
                  tunnel: w101 -> [w102 w112]
                  frame #0 {
                    n142 = case shown="True" w102 {
                      frame False {
                      }
                      frame True {
                        n143 = property on="Flow" class="DigNum (strict)"() -> ("Value"=w110:dbl)  [unwired: 2 in, 2 out]
                        n144 = property on="Calculated" class="Ring (strict)"() -> ("Value"=w111:u16)  [unwired: 2 in, 2 out]
                        n145 = property on="MFC1 flow" class="DigNum (strict)"() -> ("Value"=w109:dbl)  [unwired: 2 in, 2 out]
                        n146 = property on="MFC2 flow" class="DigNum (strict)"() -> ("Value"=w108:dbl)  [unwired: 2 in, 2 out]
                        n147 = property on="MFC3 flow" class="DigNum (strict)"() -> ("Value"=w107:dbl)  [unwired: 2 in, 2 out]
                        n148 = call "dilutionCalc.vi"("Calculated"=w111, "MFC3"=w107, "MFC2"=w108, "MFC1"=w109, "flow"=w110) -> ("MFC3 out"=w103:dbl, "MFC2 out"=w104:dbl, "MFC1 out"=w105:dbl, "flow out"=w106:dbl)  [unwired: 1 in]
                        n149 = property on="MFC1 flow" class="DigNum (strict)"("Value"=w105) -> ()  [unwired: 2 in, 2 out]
                        n150 = property on="Flow" class="DigNum (strict)"("Value"=w106) -> ()  [unwired: 2 in, 2 out]
                        n151 = property on="MFC3 flow" class="DigNum (strict)"("Value"=w103) -> ()  [unwired: 2 in, 2 out]
                        n152 = property on="MFC2 flow" class="DigNum (strict)"("Value"=w104) -> ()  [unwired: 2 in, 2 out]
                      }
                    }
                  }
                  frame #1 {
                    n153 = case shown="False" w112 {
                      frame False {
                        n154 = property on="Flow" class="DigNum (strict)"("DisabledEnum"=T15."Enabled" ("Disabled")) -> ()  [unwired: 2 in, 2 out]
                      }
                      frame True {
                        n155 = property on="Calculated" class="Ring (strict)"() -> ("Value"=w114:u16)  [unwired: 2 in, 2 out]
                        n156 = call "DilutionVisible.vi"("calculated"=w114) -> ("MFC3"=w118:u16, "MFC2"=w117:u16, "MFC1"=w116:u16, "flow"=w115:u16)  [unwired: 3 in]
                        n157 = property on="MFC1 flow" class="DigNum (strict)"("DisabledEnum"=w116) -> ()  [unwired: 2 in, 2 out]
                        n158 = property on="MFC2 flow" class="DigNum (strict)"("DisabledEnum"=w117) -> ()  [unwired: 2 in, 2 out]
                        n159 = property on="MFC3 flow" class="DigNum (strict)"("DisabledEnum"=w118) -> ()  [unwired: 2 in, 2 out]
                        n160 = property on="Flow" class="DigNum (strict)"("DisabledEnum"=w115) -> ()  [unwired: 2 in, 2 out]
                      }
                    }
                    n161 = property on="Calculated" class="Ring (strict)"("Visible"=w112) -> ()  [unwired: 2 in, 2 out]
                    n162 = property on="MFC1 flow" class="DigNum (strict)"("Visible"=w112) -> ()  [unwired: 2 in, 2 out]
                    n163 = property on="MFC2 flow" class="DigNum (strict)"("Visible"=w112) -> ()  [unwired: 2 in, 2 out]
                    n164 = property on="MFC3 flow" class="DigNum (strict)"("Visible"=w112) -> ()  [unwired: 2 in, 2 out]
                  }
                }
              }
              event Value Change {
                n165 = event-data() -> ()  [unwired: 1 in, 5 out]
                n166 = property on="Dilution" class="Bool (strict)"() -> ("Value"=w119:bool)  [unwired: 2 in, 2 out]
                n167 = stacked-sequence {
                  tunnel: w119 -> [w120 w130]
                  frame #0 {
                    n168 = case shown="True" w120 {
                      frame False {
                      }
                      frame True {
                        n169 = property on="Flow" class="DigNum (strict)"() -> ("Value"=w128:dbl)  [unwired: 2 in, 2 out]
                        n170 = property on="Calculated" class="Ring (strict)"() -> ("Value"=w129:u16)  [unwired: 2 in, 2 out]
                        n171 = property on="MFC1 flow" class="DigNum (strict)"() -> ("Value"=w127:dbl)  [unwired: 2 in, 2 out]
                        n172 = property on="MFC2 flow" class="DigNum (strict)"() -> ("Value"=w126:dbl)  [unwired: 2 in, 2 out]
                        n173 = property on="MFC3 flow" class="DigNum (strict)"() -> ("Value"=w125:dbl)  [unwired: 2 in, 2 out]
                        n174 = call "dilutionCalc.vi"("Calculated"=w129, "MFC3"=w125, "MFC2"=w126, "MFC1"=w127, "flow"=w128) -> ("MFC3 out"=w121:dbl, "MFC2 out"=w122:dbl, "MFC1 out"=w123:dbl, "flow out"=w124:dbl)  [unwired: 1 in]
                        n175 = property on="MFC1 flow" class="DigNum (strict)"("Value"=w123) -> ()  [unwired: 2 in, 2 out]
                        n176 = property on="Flow" class="DigNum (strict)"("Value"=w124) -> ()  [unwired: 2 in, 2 out]
                        n177 = property on="MFC3 flow" class="DigNum (strict)"("Value"=w121) -> ()  [unwired: 2 in, 2 out]
                        n178 = property on="MFC2 flow" class="DigNum (strict)"("Value"=w122) -> ()  [unwired: 2 in, 2 out]
                      }
                    }
                  }
                  frame #1 {
                    n179 = case shown="True" w130 {
                      frame False {
                        n180 = property on="Flow" class="DigNum (strict)"("DisabledEnum"=T15."Enabled" ("Disabled")) -> ()  [unwired: 2 in, 2 out]
                      }
                      frame True {
                        n181 = property on="Calculated" class="Ring (strict)"() -> ("Value"=w132:u16)  [unwired: 2 in, 2 out]
                        n182 = call "DilutionVisible.vi"("calculated"=w132) -> ("MFC3"=w136:u16, "MFC2"=w135:u16, "MFC1"=w134:u16, "flow"=w133:u16)  [unwired: 3 in]
                        n183 = property on="MFC1 flow" class="DigNum (strict)"("DisabledEnum"=w134) -> ()  [unwired: 2 in, 2 out]
                        n184 = property on="MFC2 flow" class="DigNum (strict)"("DisabledEnum"=w135) -> ()  [unwired: 2 in, 2 out]
                        n185 = property on="MFC3 flow" class="DigNum (strict)"("DisabledEnum"=w136) -> ()  [unwired: 2 in, 2 out]
                        n186 = property on="Flow" class="DigNum (strict)"("DisabledEnum"=w133) -> ()  [unwired: 2 in, 2 out]
                      }
                    }
                    n187 = property on="Calculated" class="Ring (strict)"("Visible"=w130) -> ()  [unwired: 2 in, 2 out]
                    n188 = property on="MFC1 flow" class="DigNum (strict)"("Visible"=w130) -> ()  [unwired: 2 in, 2 out]
                    n189 = property on="MFC2 flow" class="DigNum (strict)"("Visible"=w130) -> ()  [unwired: 2 in, 2 out]
                    n190 = property on="MFC3 flow" class="DigNum (strict)"("Visible"=w130) -> ()  [unwired: 2 in, 2 out]
                  }
                }
              }
            }
          }
        }
        frame #2 {
          n191 = property on="is OK?" class="Bool (strict)"() -> ("Value"=w137:bool)  [unwired: 2 in, 2 out]
          n192 = Not(x=w137) -> (.not. x?=w141:bool)
          n193 = Current VI's Path() -> (path=w140:path)
          n194 = call "API_Edit.vi"("Cancel"=w141, "OK"=w137, "VI Path"=w140, "Argument List In"=w138) -> ("Argument List Out"=w139:string[])
        }
      }
      n195 = property class="VI"(reference=w22, "Front Panel.Open"=FALSE ("Front Panel Window:Open"), "FP.Behavior"=T14."Default" ("Front Panel Window:Behavior")) -> (reference out=w23:refnum<vi>)  [unwired: 1 in, 1 out]
      n196 = Close Reference(reference=w23) -> ()  [unwired: 1 in, 1 out]
    }
    frame "Start" {
      n197 = call "Set_Argument.vi"("Enable"=FALSE, "Argument"="run_started", "Argument List In"=w148) -> ("Argument List Out"=w147:string[])
      n198 = property on="prep_time" class="DigNum (strict)"() -> ("Value"=w146:dbl)  [unwired: 2 in, 2 out]
      n199 = Greater Than 0?(x=w146) -> (x > 0?=w145:bool)
      n200 = Not(x=w143) -> (.not. x?=w142:bool)
      n201 = And(x=w142, y=w145) -> (x .and. y?=w144:bool)
      n202 = case shown="True" w144 {
        frame False {
        }
        frame True {
          n203 = property on="In bubbler" class="Clust (strict)"() -> ("Value"=w156:T8)  [unwired: 2 in, 2 out]
          n204 = property on="Ga bubbler" class="Clust (strict)"() -> ("Value"=w157:T16)  [unwired: 2 in, 2 out]
          n205 = property on="Al bubbler" class="Clust (strict)"() -> ("Value"=w158:T11)  [unwired: 2 in, 2 out]
          n206 = property on="Se bubbler" class="Clust (strict)"() -> ("Value"=w151:T16)  [unwired: 2 in, 2 out]
          n207 = property on="P bubbler" class="Clust (strict)"() -> ("Value"=w153:T2)  [unwired: 2 in, 2 out]
          n208 = property on="P gas" class="Clust (strict)"() -> ("Value"=w155:T6)  [unwired: 2 in, 2 out]
          n209 = property on="As gas" class="Clust (strict)"() -> ("Value"=w154:T4)  [unwired: 2 in, 2 out]
          n210 = call "Set_V_III.vi"("Se bubbler"=w151, "P bubbler"=w153, "As gas"=w154, "P gas"=w155, "Run Started"=FALSE, "In bubbler"=w156, "Ga bubbler"=w157, "Al bubbler"=w158) -> ()  [unwired: 4 in]
        }
      }
    }
    frame "Run" {
      n211 = stacked-sequence {
        tunnel: w162 -> [_ w167 _ _]
        tunnel: w160 -> [w164 _ _ w248]
        tunnel: w161 -> [_ _ _ w246]
        tunnel: [_ _ _ w247] -> w159
        frame #0 {
          n212 = call "Get_Argument.vi"("Argument"="run_started", "Argument List"=w164) -> ("Enabled"=w163:bool)
          n213 = local write "run started"(w163) -> ()
        }
        frame #1 {
          n214 = property on="prep_time" class="DigNum (strict)"() -> ("Value"=w168:dbl)  [unwired: 2 in, 2 out]
          n215 = Greater Or Equal?(x=w167, y=w168) -> (x >= y?=w166:bool)
          n216 = local write "prep_done"(w166) -> ()
        }
        frame #2 {
          n217 = local read "run started"() -> (w170:bool)
          n218 = Not(x=w170) -> (.not. x?=w169:bool)
          n219 = stacked-sequence {
            tunnel: w169 -> [w172 w179 w189 w199 w209 w219 w229 w239]
            frame #0 {
              n220 = case shown="False" w172 {
                tunnel: ["run: " "pre-run: "] -> w171
                frame False {
                }
                frame True {
                }
              }
              n221 = property on="Status Out" class="Str"("Value"=w171) -> ()  [unwired: 2 in, 2 out]
            }
            frame #1 {
              n222 = property on="Al main" class="Clust (strict)"() -> ("Value"=w177:T17)  [unwired: 2 in, 2 out]
              n223 = property on="Al Active" class="Bool (strict)"() -> ("Value"=w178:bool)  [unwired: 2 in, 2 out]
              n224 = property on="Status Out" class="Str"() -> ("Value"=w184:string)  [unwired: 2 in, 2 out]
              n225 = Unbundle By Name(w177) -> ("Al Run"=w176:bool, "Prep Al"=w175:bool)
              n226 = call "flow_strings.vi"("string in"=w184, "is first in?"=TRUE, "use source?"=w178, "name"="Al", "run source?"=w176, "prep source?"=w175, "is prep?"=w179) -> ("string out"=w183:string, "is first out?"=w182:bool)
              n227 = property on="Status Out" class="Str"("Value"=w183) -> ()  [unwired: 2 in, 2 out]
              n228 = property on="first" class="Bool (strict)"("Value"=w182) -> ()  [unwired: 2 in, 2 out]
            }
            frame #2 {
              n229 = property on="main" class="Clust (strict)"() -> ("Value"=w187:T18)  [unwired: 2 in, 2 out]
              n230 = property on="Active" class="Bool (strict)"() -> ("Value"=w188:bool)  [unwired: 2 in, 2 out]
              n231 = property on="first" class="Bool (strict)"() -> ("Value"=w191:bool)  [unwired: 2 in, 2 out]
              n232 = property on="Status Out" class="Str"() -> ("Value"=w193:string)  [unwired: 2 in, 2 out]
              n233 = Unbundle By Name(w187) -> ("Run"=w186:bool, "Prep Ga"=w185:bool)
              n234 = call "flow_strings.vi"("string in"=w193, "is first in?"=w191, "use source?"=w188, "name"="Ga", "run source?"=w186, "prep source?"=w185, "is prep?"=w189) -> ("string out"=w194:string, "is first out?"=w190:bool)
              n235 = property on="Status Out" class="Str"("Value"=w194) -> ()  [unwired: 2 in, 2 out]
              n236 = property on="first" class="Bool (strict)"("Value"=w190) -> ()  [unwired: 2 in, 2 out]
            }
            frame #3 {
              n237 = property on="In bubbler Active" class="Bool (strict)"() -> ("Value"=w198:bool)  [unwired: 2 in, 2 out]
              n238 = property on="In main" class="Clust (strict)"() -> ("Value"=w197:T19)  [unwired: 2 in, 2 out]
              n239 = property on="first" class="Bool (strict)"() -> ("Value"=w202:bool)  [unwired: 2 in, 2 out]
              n240 = property on="Status Out" class="Str"() -> ("Value"=w204:string)  [unwired: 2 in, 2 out]
              n241 = Unbundle By Name(w197) -> ("In Run"=w196:bool, "Prep In"=w195:bool)
              n242 = call "flow_strings.vi"("string in"=w204, "is first in?"=w202, "use source?"=w198, "name"="In", "run source?"=w196, "prep source?"=w195, "is prep?"=w199) -> ("string out"=w201:string, "is first out?"=w200:bool)
              n243 = property on="Status Out" class="Str"("Value"=w201) -> ()  [unwired: 2 in, 2 out]
              n244 = property on="first" class="Bool (strict)"("Value"=w200) -> ()  [unwired: 2 in, 2 out]
            }
            frame #4 {
              n245 = property on="P gas Active" class="Bool (strict)"() -> ("Value"=w208:bool)  [unwired: 2 in, 2 out]
              n246 = property on="P gas main" class="Clust (strict)"() -> ("Value"=w207:T20)  [unwired: 2 in, 2 out]
              n247 = property on="first" class="Bool (strict)"() -> ("Value"=w211:bool)  [unwired: 2 in, 2 out]
              n248 = property on="Status Out" class="Str"() -> ("Value"=w213:string)  [unwired: 2 in, 2 out]
              n249 = Unbundle By Name(w207) -> ("PH3 Run"=w206:bool, "PH3 Prep"=w205:bool)
              n250 = call "flow_strings.vi"("string in"=w213, "is first in?"=w211, "use source?"=w208, "name"="PH3", "run source?"=w206, "prep source?"=w205, "is prep?"=w209) -> ("string out"=w212:string, "is first out?"=w210:bool)
              n251 = property on="Status Out" class="Str"("Value"=w212) -> ()  [unwired: 2 in, 2 out]
              n252 = property on="first" class="Bool (strict)"("Value"=w210) -> ()  [unwired: 2 in, 2 out]
            }
            frame #5 {
              n253 = property on="As gas Active" class="Bool (strict)"() -> ("Value"=w218:bool)  [unwired: 2 in, 2 out]
              n254 = property on="As gas main" class="Clust (strict)"() -> ("Value"=w217:T21)  [unwired: 2 in, 2 out]
              n255 = property on="first" class="Bool (strict)"() -> ("Value"=w221:bool)  [unwired: 2 in, 2 out]
              n256 = property on="Status Out" class="Str"() -> ("Value"=w223:string)  [unwired: 2 in, 2 out]
              n257 = Unbundle By Name(w217) -> ("AsH3 Run"=w216:bool, "AsH3 Prep"=w215:bool)
              n258 = call "flow_strings.vi"("string in"=w223, "is first in?"=w221, "use source?"=w218, "name"="AsH3", "run source?"=w216, "prep source?"=w215, "is prep?"=w219) -> ("string out"=w220:string, "is first out?"=w222:bool)
              n259 = property on="Status Out" class="Str"("Value"=w220) -> ()  [unwired: 2 in, 2 out]
              n260 = property on="first" class="Bool (strict)"("Value"=w222) -> ()  [unwired: 2 in, 2 out]
            }
            frame #6 {
              n261 = property on="P bubbler main" class="Clust (strict)"() -> ("Value"=w227:T22)  [unwired: 2 in, 2 out]
              n262 = property on="P bubbler Active" class="Bool (strict)"() -> ("Value"=w228:bool)  [unwired: 2 in, 2 out]
              n263 = Unbundle By Name(w227) -> ("P bubbler Run"=w226:bool, "P bubbler Prep"=w225:bool)
              n264 = property on="first" class="Bool (strict)"() -> ("Value"=w232:bool)  [unwired: 2 in, 2 out]
              n265 = property on="Status Out" class="Str"() -> ("Value"=w234:string)  [unwired: 2 in, 2 out]
              n266 = call "flow_strings.vi"("string in"=w234, "is first in?"=w232, "use source?"=w228, "name"="P liq", "run source?"=w226, "prep source?"=w225, "is prep?"=w229) -> ("string out"=w231:string, "is first out?"=w230:bool)
              n267 = property on="Status Out" class="Str"("Value"=w231) -> ()  [unwired: 2 in, 2 out]
              n268 = property on="first" class="Bool (strict)"("Value"=w230) -> ()  [unwired: 2 in, 2 out]
            }
            frame #7 {
              n269 = property on="main" class="Clust (strict)"() -> ("Value"=w237:T18)  [unwired: 2 in, 2 out]
              n270 = property on="Active" class="Bool (strict)"() -> ("Value"=w238:bool)  [unwired: 2 in, 2 out]
              n271 = property on="first" class="Bool (strict)"() -> ("Value"=w242:bool)  [unwired: 2 in, 2 out]
              n272 = property on="Status Out" class="Str"() -> ("Value"=w244:string)  [unwired: 2 in, 2 out]
              n273 = Unbundle By Name(w237) -> ("Run"=w236:bool, "Prep Ga"=w235:bool)
              n274 = call "flow_strings.vi"("string in"=w244, "is first in?"=w242, "use source?"=w238, "name"="Se", "run source?"=w236, "prep source?"=w235, "is prep?"=w239) -> ("string out"=w241:string, "is first out?"=w240:bool)
              n275 = property on="Status Out" class="Str"("Value"=w241) -> ()  [unwired: 2 in, 2 out]
              n276 = property on="first" class="Bool (strict)"("Value"=w240) -> ()  [unwired: 2 in, 2 out]
            }
          }
        }
        frame #3 {
          n277 = property on="prep_done" class="Bool (strict)"() -> ("Value"=w251:bool)  [unwired: 2 in, 2 out]
          n278 = property on="run started" class="Bool (strict)"() -> ("Value"=w250:bool)  [unwired: 2 in, 2 out]
          n279 = Not(x=w250) -> (.not. x?=w249:bool)
          n280 = And(x=w251, y=w249) -> (x .and. y?=w245:bool)
          n281 = case shown="True" w245 {
            selector: w245 -> [_ w253]
            tunnel: w248 -> [w252 w256]
            tunnel: [w252 w255] -> w247
            tunnel: w246 -> [_ w254]
            frame False {
            }
            frame True {
              n282 = stacked-sequence {
                tunnel: w254 -> [w258 _]
                tunnel: w256 -> [_ w268]
                tunnel: [_ w267] -> w255
                tunnel: w253 -> [w257 _]
                frame #0 {
                  n283 = case shown="False" w258 {
                    tunnel: w257 -> [w260 _]
                    frame False {
                      n284 = property on="In bubbler" class="Clust (strict)"() -> ("Value"=w264:T8)  [unwired: 2 in, 2 out]
                      n285 = property on="Ga bubbler" class="Clust (strict)"() -> ("Value"=w265:T16)  [unwired: 2 in, 2 out]
                      n286 = property on="Al bubbler" class="Clust (strict)"() -> ("Value"=w266:T11)  [unwired: 2 in, 2 out]
                      n287 = property on="Se bubbler" class="Clust (strict)"() -> ("Value"=w259:T16)  [unwired: 2 in, 2 out]
                      n288 = property on="P gas" class="Clust (strict)"() -> ("Value"=w263:T6)  [unwired: 2 in, 2 out]
                      n289 = property on="As gas" class="Clust (strict)"() -> ("Value"=w262:T4)  [unwired: 2 in, 2 out]
                      n290 = property on="P bubbler" class="Clust (strict)"() -> ("Value"=w261:T2)  [unwired: 2 in, 2 out]
                      n291 = call "Set_V_III.vi"("Se bubbler"=w259, "P bubbler"=w261, "As gas"=w262, "P gas"=w263, "Run Started"=w260, "In bubbler"=w264, "Ga bubbler"=w265, "Al bubbler"=w266) -> ()  [unwired: 4 in]
                    }
                    frame True {
                    }
                  }
                }
                frame #1 {
                  n292 = call "Set_Argument.vi"("Enable"=TRUE, "Argument"="run_started", "Argument List In"=w268) -> ("Argument List Out"=w267:string[])
                }
              }
            }
          }
        }
      }
    }
    frame "End" {
    }
    frame "Idle" {
    }
  }
  "Argument List Out" <- w10
